vi "DropAndCreateString.vi"(10 "Items":string[](array[string])=["C1", "C2", "C3"], 11 "Table Name":string="temp") -> (3 "Drop and Create String":string)   [LabVIEW 2015, in "DBToolkit.lvlib"]
uses:
  DBToolkit.lvlib
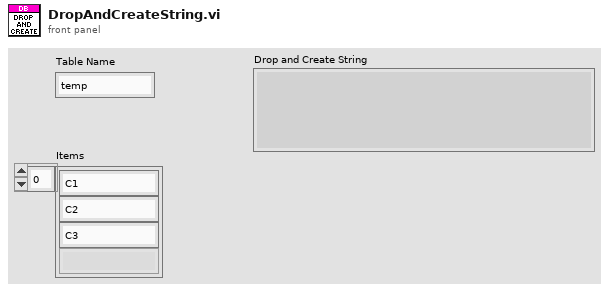
[diagram p1: front panel]
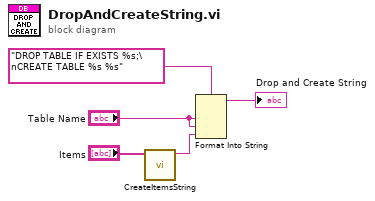
[diagram p0: block diagram]
diagram:
  n1 = call "CreateItemsString.vi"("Items"="Items") -> ("Items for CREATE"=w3:string)  [unwired: 8 in, 2 out]
  n2 = Format Into String(format string="DROP TABLE IF EXISTS %s;\nCREATE TABLE %s %s" ("string"), "Table Name", "Table Name", w3) -> (resulting string=→"Drop and Create String":string)  [unwired: 2 in, 1 out]
